vi "2D DCT.vi"(11 "X":dbl[][](array[numeric])) -> (0 "error":i32, 3 "DCT {X}":dbl[][](array[numeric]))   [LabVIEW 2020, in "NI_AALPro.lvlib"]
doc: "Computes the Discrete Cosine Transform (DCT) of the input sequence <B>X</B>. Wire data to the <B>X</B> input to determine the polymorphic instance to use or manually select the instance."
uses:
  NI_AALPro.lvlib
  <resource>/lvanlys.dll
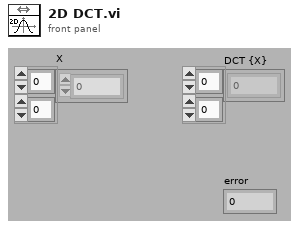
[diagram p1: front panel]
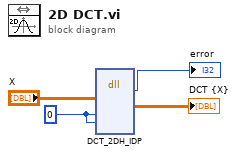
[diagram p0: block diagram]
diagram:
  w1 = 0 ("m")
  n1 = dll-call lib="C:/Program Files (x86)/National Instruments/LabVIEW 2020/resource/lvanlys.*" fn="DCT_2DH_IDP"("xH"="X", "m"=w1, "n"=w1) -> ("return type"=→"error":i32, "yH"=→"DCT {X}":dbl[][])  [unwired: 9 in, 2 out]
